vi "Move.vi"(0 "Points":cluster{string, "data":u64, "data":dbl}[](array[cluster])=[{"0:0", "data"=0, "data"=-0.0}], 1 "Sweep inst info":T3(array[cluster])=[{"Kind"=4, "Strings"=["0:0", "192.168.0.21", "V"], "uint64s"=[0, 0], "Doubles"=[0.5, -2.0, 2.0, -1.0], "DAQmx take out list"=[]}], 2 "FPGA Ref":T2, 3 "Use FPGA?":bool=TRUE, 4 "WorkFilePath":path, 5 "Indexes":u64[](array[numeric])) -> (7 "FPGA VI Reference Out":T2)   [LabVIEW 2013]
uses:
  fpga-bitfile-ref.ctl
panel:
  out "Delay line information":T1
  out "Wait delay line":bool
  out "Wait (ms)":dbl
  out "Wait ??":bool
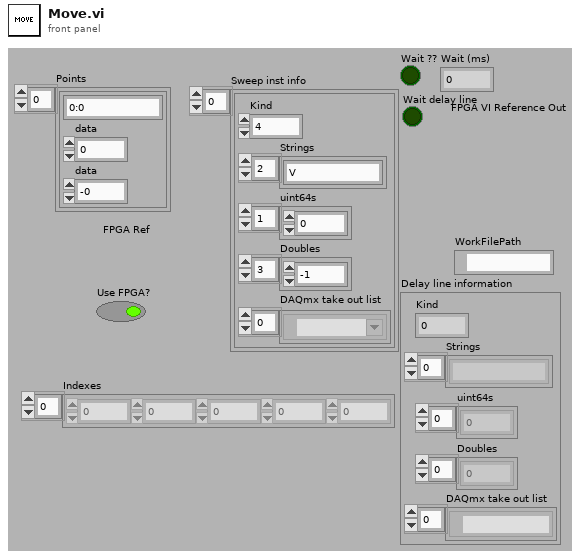
[diagram p1: front panel]
types:
  T1 = cluster{"Kind":u16, "Strings":string[], "uint64s":u64[], "Doubles":dbl[], "DAQmx take out list":refnum<k21>[]}
  T2 = typedef "fpga-bitfile-ref.ctl" = refnum<k20>
  T3 = cluster{"Kind":u16, "Strings":string[], "uint64s":u64[], "Doubles":dbl[], "DAQmx take out list":refnum<k21>[]}[]
  T4 = enum8{"start movement", "buses to use", "delay", "value", "stop", ""}
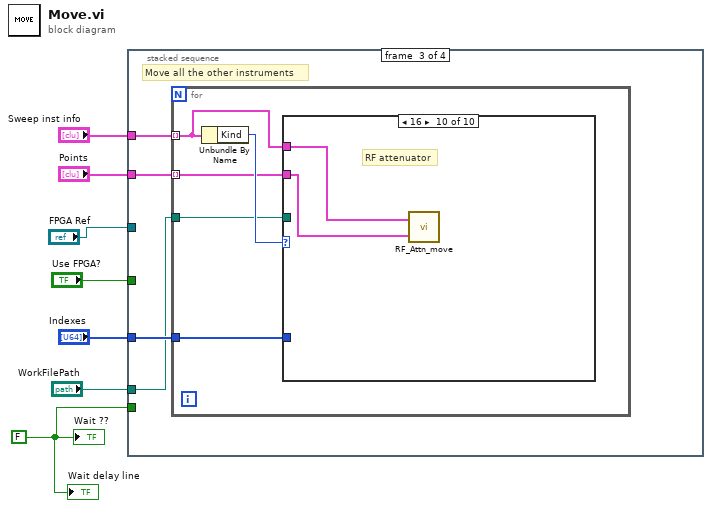
[diagram p0: block diagram]
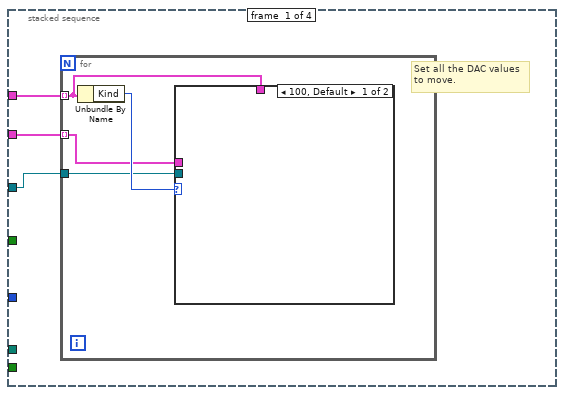
[diagram p2: hidden frame]
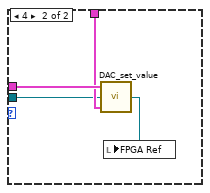
[diagram p3: hidden frame]
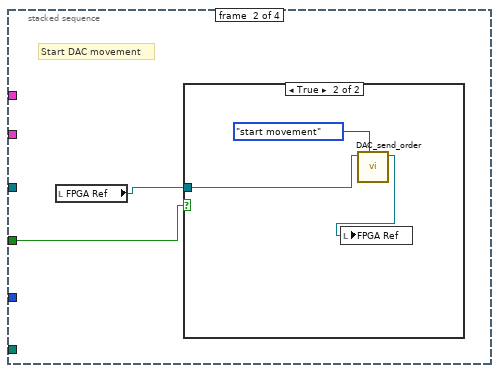
[diagram p4: hidden frame]
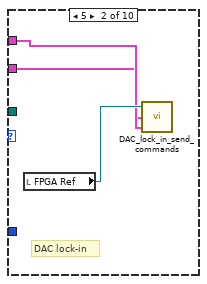
[diagram p7: hidden frame]
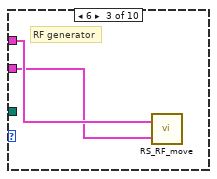
[diagram p8: hidden frame]
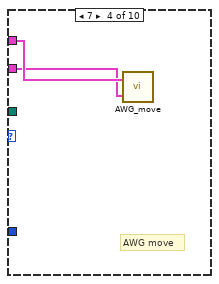
[diagram p9: hidden frame]
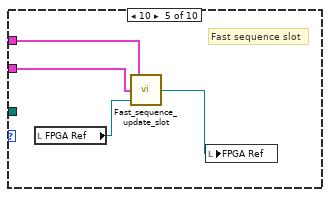
[diagram p10: hidden frame]
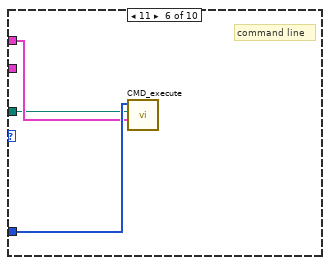
[diagram p11: hidden frame]
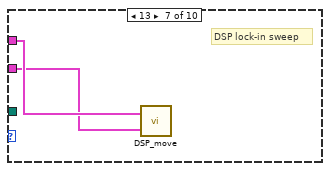
[diagram p12: hidden frame]
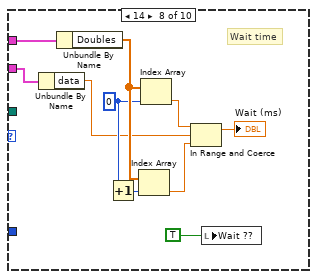
[diagram p13: hidden frame]
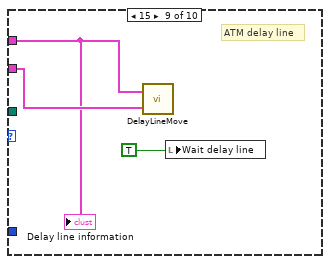
[diagram p14: hidden frame]
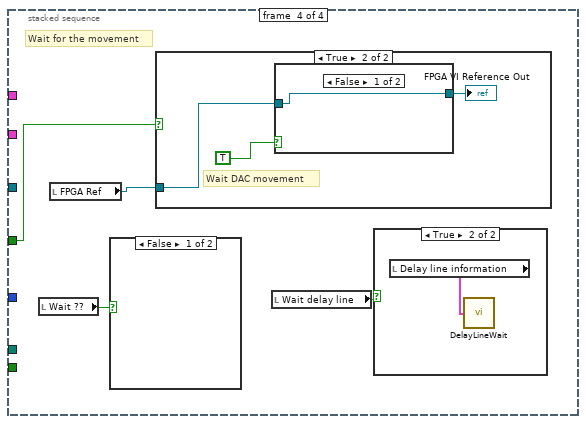
[diagram p15: hidden frame]
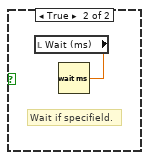
[diagram p17: hidden frame]
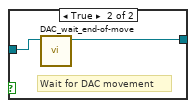
[diagram p19: hidden frame]
diagram:
  w1 = FALSE
  n1 = stacked-sequence {
    tunnel: "Sweep inst info" -> [w9 _ w27 _]
    tunnel: "Points" -> [w10 _ w26 _]
    tunnel: "Use FPGA?" -> [_ w20 _ w67]
    tunnel: "FPGA Ref" -> [w8 _ _ _]
    tunnel: "Indexes" -> [_ _ w25 _]
    tunnel: "WorkFilePath" -> [_ _ w24 _]
    tunnel: w1 -> [_ _ _ _]
    frame #0 {
      # "Set all the DAC values\nto move."
      n2 = for {
        tunnel: w10 -> [w13] mode=indexing
        tunnel: w9 -> [w12] mode=indexing
        tunnel: w8 -> [w11]
        n3 = Unbundle By Name(w12) -> ("Kind"=w14:u16)
        n4 = case shown="100, Default" w14 {
          tunnel: w13 -> [_ w18]
          tunnel: w12 -> [_ w17]
          tunnel: w11 -> [_ w16]
          frame 100, Default {
          }
          frame 4 {
            n5 = call "DAC_set_value.vi"("InstInfo"=w17, "FPGA Ref"=w16, "Point"=w18) -> ("FPGA VI Reference Out"=w15:T2)
            n6 = local write "FPGA Ref"(w15) -> ()
          }
        }
      }
    }
    frame #1 {
      # "Start DAC movement"
      n7 = local read "FPGA Ref"() -> (w19:T2)
      n8 = case shown="True" w20 {
        tunnel: w19 -> [_ w22]
        frame False {
        }
        frame True {
          n9 = call "DAC_send_order.vi"("order"=T4."start movement", "FPGA VI Reference In"=w22) -> ("FPGA VI Reference Out"=w21:T2)  [unwired: 5 in, 4 out]
          n10 = local write "FPGA Ref"(w21) -> ()
        }
      }
    }
    frame #2 {
      # "Move all the other instruments"
      n11 = for {
        tunnel: w27 -> [w31] mode=indexing
        tunnel: w26 -> [w30] mode=indexing
        tunnel: w25 -> [w29]
        tunnel: w24 -> [w28]
        n12 = Unbundle By Name(w31) -> ("Kind"=w32:u16)
        n13 = case shown="16" w32 {
          tunnel: w31 -> [_ w34 w37 w39 w42 w45 w48 w58 w60 w63]
          tunnel: w30 -> [_ w33 w36 w38 w43 _ w47 w57 w61 w62]
          tunnel: w29 -> [_ _ _ _ _ w46 _ _ _ _]
          tunnel: w28 -> [_ _ _ _ _ w44 _ _ _ _]
          frame 100, Default {
          }
          frame 5 {
            # "DAC lock-in"
            n14 = local read "FPGA Ref"() -> (w35:T2)
            n15 = call "DAC_lock_in_send_commands.vi"("Inst info"=w34, "Points"=w33, "FPGA VI Reference In"=w35) -> ()  [unwired: 1 in]
          }
          frame 6 {
            # "RF generator"
            n16 = call "RS_RF_move.vi"("Points"=w36, "Instr. Info"=w37) -> ()  [unwired: 1 in]
          }
          frame 7 {
            # "AWG move"
            n17 = call "AWG_move.vi"("Point"=w38, "inst info"=w39) -> ()  [unwired: 1 out]
          }
          frame 10 {
            # "Fast sequence slot"
            n18 = local read "FPGA Ref"() -> (w40:T2)
            n19 = call "Fast_sequence_update_slot.vi"("FPGA Ref"=w40, "Points"=w43, "Inst param"=w42) -> ("FPGA Ref Out"=w41:T2)
            n20 = local write "FPGA Ref"(w41) -> ()
          }
          frame 11 {
            # "command line"
            n21 = call "CMD_execute.vi"("Inst_info"=w45, "WorkFilePath"=w44, "Indexes"=w46) -> ()  [unwired: 2 in]
          }
          frame 13 {
            # "DSP lock-in sweep"
            n22 = call "DSP_move.vi"("Points"=w47, "Instr. Info"=w48) -> ()  [unwired: 1 in]
          }
          frame 14 {
            w55 = 0
            # "Wait time"
            n23 = Unbundle By Name(w57) -> ("data"=w51:dbl)
            n24 = Unbundle By Name(w58) -> ("Doubles"=w56:dbl[])
            n25 = Increment(x=w55) -> (x+1=w54:i32)
            n26 = Index Array(array=w56, index=w54) -> (element=w53:dbl)
            n27 = Index Array(array=w56, index=w55) -> (element=w52:dbl)
            n28 = In Range and Coerce(upper limit=w52, x=w51, lower limit=w53) -> (coerced(x)=→"Wait (ms)":dbl)  [unwired: 1 out]
            n29 = local write "Wait ??"(TRUE) -> ()
          }
          frame 15 {
            # "ATM delay line"
            n30 = call "DelayLineMove.vi"("Points"=w61, "Inst_param"=w60) -> ()  [unwired: 1 in]
            n31 = local write "Wait delay line"(TRUE) -> ()
            "Delay line information" <- w60
          }
          frame 16 {
            # "RF attenuator"
            n32 = call "RF_Attn_move.vi"("Points"=w62, "Instr. Info"=w63) -> ()  [unwired: 1 in]
          }
        }
      }
    }
    frame #3 {
      # "Wait for the movement"
      n33 = local read "Wait ??"() -> (w65:bool)
      n34 = local read "FPGA Ref"() -> (w66:T2)
      n35 = case shown="False" w65 {
        frame False {
        }
        frame True {
          # "Wait if specifield."
          n36 = local read "Wait (ms)"() -> (w69:dbl)
          n37 = Wait (ms)(milliseconds to wait=w69) -> ()  [unwired: 1 out]
        }
      }
      n38 = case shown="True" w67 {
        tunnel: w66 -> [_ w71]
        frame False {
        }
        frame True {
          # "Wait DAC movement"
          n39 = case shown="False" TRUE ("Wait DAC movement") {
            tunnel: [w73 w75] -> w70
            tunnel: w71 -> [w73 w74]
            frame False {
            }
            frame True {
              # "Wait for DAC movement"
              n40 = call "DAC_wait_end-of-move.vi"("FPGA VI Reference In"=w74) -> ("FPGA VI Reference Out"=w75:T2)  [unwired: 10 out]
            }
          }
          "FPGA VI Reference Out" <- w70
        }
      }
      n41 = local read "Wait delay line"() -> (w64:bool)
      n42 = case shown="True" w64 {
        frame False {
        }
        frame True {
          n43 = local read "Delay line information"() -> (w68:T1)
          n44 = call "DelayLineWait.vi"("Inst_param"=w68) -> ()
        }
      }
    }
  }
  "Wait ??" <- w1
  "Wait delay line" <- w1
